vi "ClearBus.vi"(8 "ErrorIn":errorcluster[](array[cluster])) -> (0 "ErrorOut":errorcluster[](array[cluster]))   [LabVIEW 2018, in "Bus.lvclass"]
uses:
  Bus.lvclass
  Bus.lvclass/Bus.ctl
  Accessors/Read BusNumber.vi
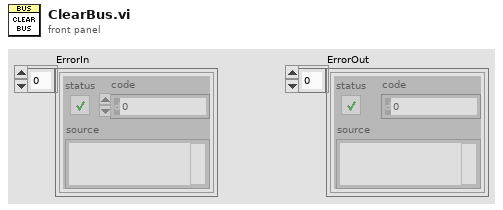
[diagram p1: front panel]
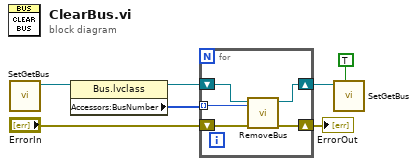
[diagram p0: block diagram]
diagram:
  n1 = call "SetGetBus.vi"() -> ("Bus.lvclass"=w5:refnum<class "Bus.lvclass">)  [unwired: 11 in]
  n2 = property class="Bus.lvclass"(reference=w5) -> (reference out=w7:refnum<class "Bus.lvclass">, "Accessors:BusNumber"=w3:i32[])  [unwired: 1 in, 1 out]
  n3 = for {
    shift-right: [w11] -> w1
    shift-left: "ErrorIn" -> [w12]
    shift-right: [w8] -> w6
    shift-left: w7 -> [w10]
    tunnel: w3 -> [w9] mode=indexing
    n4 = call "RemoveBus.vi"("BusNumber"=w9, "ErrorIn"=w12, "Bus.lvclass"=w10) -> ("ErrorOut"=w11:errorcluster[], "Bus.lvclass"=w8:refnum<class "Bus.lvclass">)  [unwired: 7 in]
  }
  "ErrorOut" <- w1
  n5 = call "SetGetBus.vi"("Set (f)"=TRUE, "Bus.lvclass"=w6) -> ()  [unwired: 9 in, 1 out]
